vi "CAPTH-Test Stop Condition.vi"(0 "Abort?":bool, 11 "error in (no error)":errorcluster) -> (8 "Stop?":bool, 15 "error out":errorcluster)   [LabVIEW 2020]
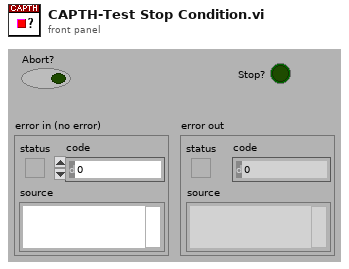
[diagram p1: front panel]
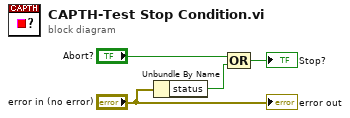
[diagram p0: block diagram]
diagram:
  n1 = Unbundle By Name("error in (no error)") -> ("status"=w3:bool)
  n2 = Compound Arithmetic op=OR("Abort?", w3) -> (→"Stop?":bool)
  "error out" <- "error in (no error)"
